vi "setVSource.vi"(8 "error in (no error)":errorcluster, 10 "Volt":i32 min=-1000 max=1000, 11 "Electrometer in":refnum<class "Electrometer.lvclass">) -> (0 "error out":errorcluster, 3 "Electrometer out":refnum<class "Electrometer.lvclass">)   [LabVIEW 2016, in "Electrometer.lvclass"]
uses:
  Electrometer.lvclass
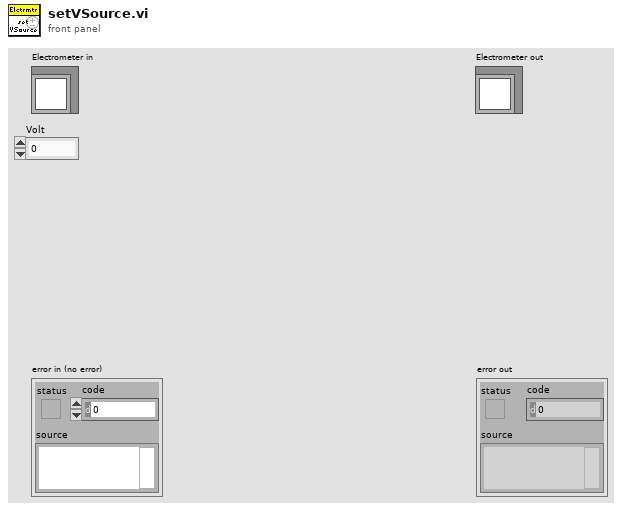
[diagram p1: front panel]
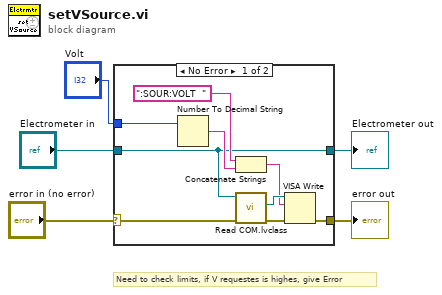
[diagram p0: block diagram]
diagram:
  # "Need to check limits, if V requestes is highes, give Error"
  n1 = case shown="No Error" "error in (no error)" {
    selector: "error in (no error)" -> [w13 w16]
    tunnel: [w14 w16] -> w4
    tunnel: [w6 w15] -> w2
    tunnel: "Electrometer in" -> [w6 w15]
    tunnel: "Volt" -> [w9 _]
    frame No Error {
      n2 = Number To Decimal String(number=w9) -> (decimal integer string=w8:string)  [unwired: 1 in]
      n3 = Concatenate Strings(":SOUR:VOLT  " ("string"), w8) -> (w7:string)
      n4 = call "Read COM.lvclass.vi"("error in (no error)"=w13, "Electrometer in"=w6) -> ("error out"=w11:errorcluster, "VISA"=w12:refnum<visa-resource-name>)  [unwired: 7 in, 1 out]
      n5 = VISA Write(VISA resource name=w12, write buffer=w7, error in (no error)=w11) -> (error out=w14:errorcluster)  [unwired: 2 out]
    }
    frame Error {
    }
  }
  "error out" <- w4
  "Electrometer out" <- w2
